vi "ReadIVBuffers.vi"(7 "GetCapacitors":bool, 8 "error in (no error)":errorcluster, 9 "Status":refnum<vi>, 10 "XYGraph Refnum":refnum<vi>, 11 "VISA Refnum in":refnum<visa-resource-name>) -> (0 "error out":errorcluster, 2 "CapacitanceInfos":T1[](array[typedef]), 3 "Array":dbl[][](array[numeric]))   [LabVIEW 2020]
uses:
  CapacitanceRecord.ctl
  Keithley 2600 Series/Keithley 2600 Series.lvlib
panel:
  out "Array 2":string[](array[string])
  out "error out 2":errorcluster
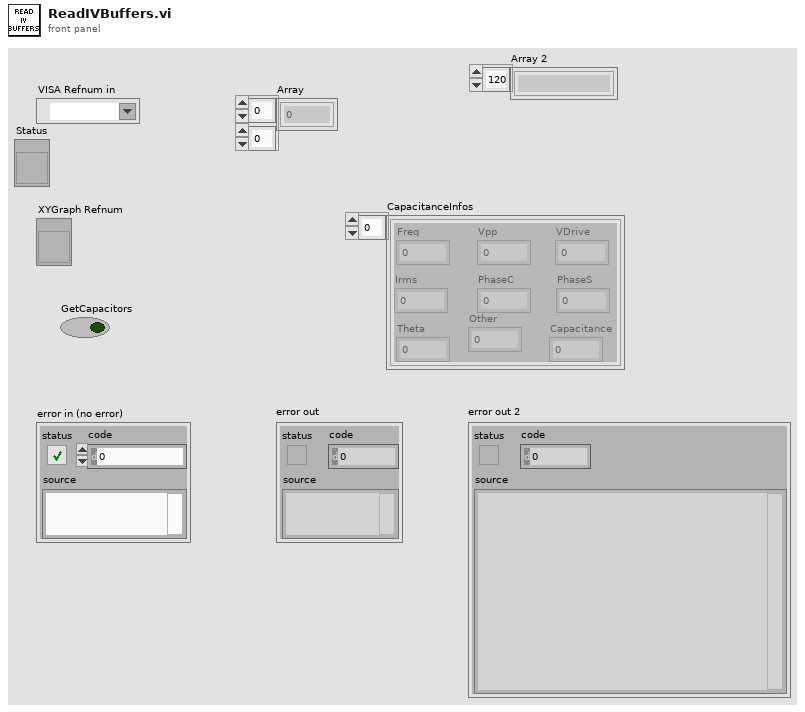
[diagram p1: front panel]
types:
  T1 = typedef "CapacitanceRecord.ctl" = cluster{"Freq":dbl, "Vpp":dbl, "PhaseS":dbl, "Irms":dbl, "PhaseC":dbl, "Theta":dbl, "VDrive":dbl, "Capacitance":dbl, "Other":dbl}
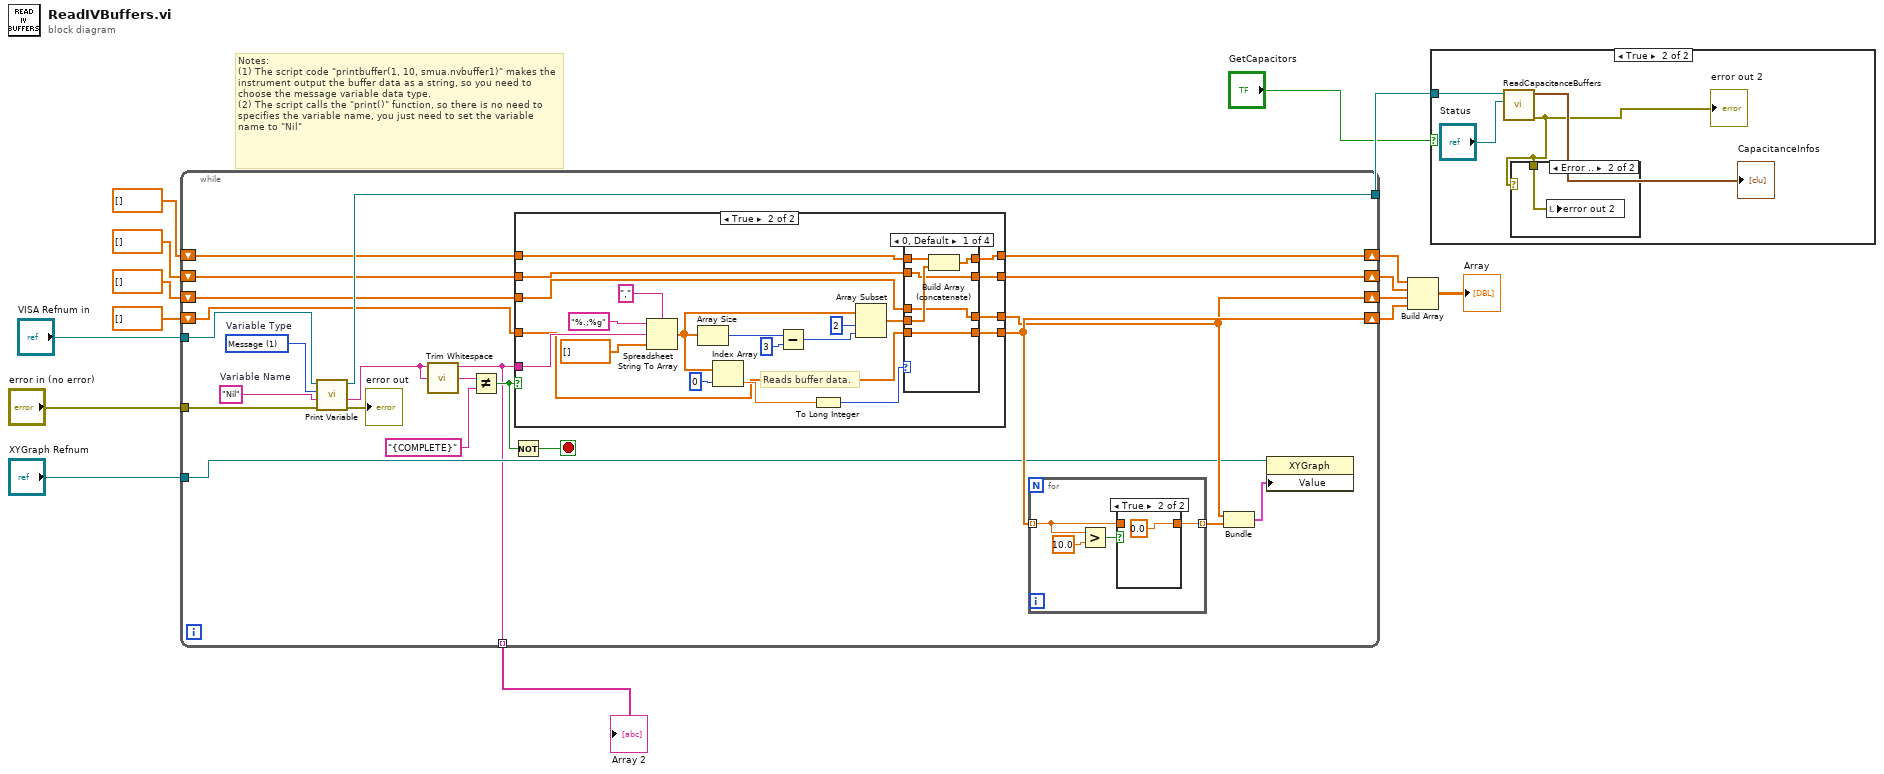
[diagram p0: block diagram]
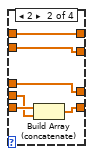
[diagram p6: hidden frame]
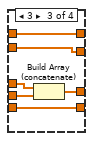
[diagram p7: hidden frame]
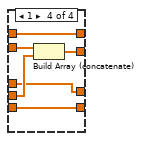
[diagram p8: hidden frame]
diagram:
  # "Notes: \n(1) The script code \"printbuffer(1, 10, smua.nvbuffer1)\" makes the instrument output the buffer data as a string, so you need to choose the message variable data type.\n(2) The script calls the \"print()\" function, so there is no need to specifies the variable name, you just need to set the variable name to \"Nil\""
  n1 = while {
    tunnel: "VISA Refnum in" -> [w35]
    tunnel: [w33] -> w3
    shift-right: [w28] -> w10
    shift-left: dbl[] [] ("array type (2D Dbl)") -> [w29]
    shift-right: [w18] -> w12
    shift-left: dbl[] [] ("array type (2D Dbl)") -> [w27]
    shift-right: [w32] -> w9
    shift-left: dbl[] [] ("array type (2D Dbl)") -> [w31]
    shift-right: [w19] -> w13
    shift-left: dbl[] [] ("array type (2D Dbl)") -> [w30]
    tunnel: "error in (no error)" -> [w22]
    tunnel: "XYGraph Refnum" -> [w17]
    tunnel: [w16] -> w1 mode=indexing
    stop <- w23 stop-if-true
    w37 = 1 items=["Number", "Message"]  # Variable Type
    w36 = "Nil"  # Variable Name
    n2 = call "Print Variable.vi"("error in (no error)"=w22, "Variable Name"=w36, "Variable Type (0: Number)"=w37, "VISA resource name"=w35) -> ("error out"=→"error out":errorcluster, "Message"=w16:string, "VISA resource name out"=w33:refnum<visa-resource-name>)  [unwired: 4 in, 1 out]
    n3 = call <vilib>:"Trim Whitespace.vi"("string"=w16) -> ("trimmed string"=w26:string)  [unwired: 1 in]
    n4 = Not Equal?(x=w26, y="{COMPLETE}") -> (x != y?=w24:bool)
    n5 = Not(x=w24) -> (.not. x?=w23:bool)
    n6 = case shown="True" w24 {
      tunnel: w16 -> [_ w65]
      tunnel: [w47 w63] -> w32
      tunnel: w31 -> [w47 w62]
      tunnel: [w45 w60] -> w19
      tunnel: w30 -> [w45 w58]
      tunnel: w29 -> [w46 w57]
      tunnel: [w46 w56] -> w28
      tunnel: w27 -> [w44 w55]
      tunnel: [w44 w54] -> w18
      frame False {
      }
      frame True {
        # "Reads buffer data."
        n7 = Spreadsheet String To Array(delimiter (Tab)=",", format string="%.;%g", spreadsheet string=w65, array type (2D Dbl)=dbl[] []) -> (array=w51:dbl[])
        n8 = Array Size(array=w51) -> (size(s)=w50:i32)
        n9 = Index Array(array=w51, index=0) -> (element=w61:dbl)
        n10 = Subtract(x=w50, y=3) -> (x-y=w48:i32)
        n11 = To Long Integer(number=w61) -> (32bit integer=w59:i32)
        n12 = Array Subset(array=w51, index=2, length=w48) -> (w53:dbl[])
        n13 = case shown="0, Default" w59 {
          tunnel: [w72 w80 w86 w92] -> w63
          tunnel: w62 -> [w74 w80 w86 w92]
          tunnel: [w71 w75 w85 w88] -> w60
          tunnel: w53 -> [w73 w78 w82 w90]
          tunnel: w58 -> [w71 w79 w85 w88]
          tunnel: w57 -> [w70 w77 w84 w91]
          tunnel: [w70 w77 w84 w89] -> w56
          tunnel: w55 -> [w69 w76 w83 w87]
          tunnel: [w69 w76 w81 w87] -> w54
          frame 0, Default {
            n14 = Build Array (concatenate)(w74, w73) -> (w72:dbl[])
          }
          frame 2 {
            n15 = Build Array (concatenate)(w79, w78) -> (w75:dbl[])
          }
          frame 3 {
            n16 = Build Array (concatenate)(w83, w82) -> (w81:dbl[])
          }
          frame 1 {
            n17 = Build Array (concatenate)(w91, w90) -> (w89:dbl[])
          }
        }
      }
    }
    n18 = for {
      tunnel: w19 -> [w39] mode=indexing
      tunnel: [w40] -> w20 mode=indexing
      n19 = Greater?(x=w39, y=10.0) -> (0:w41:bool)
      n20 = case shown="True" w41 {
        tunnel: [w42 0.0] -> w40
        tunnel: w39 -> [w42 _]
        frame False {
        }
        frame True {
        }
      }
    }
    n21 = Bundle("array type (2D Dbl)"=w18, w20) -> (w21:cluster{"array type (2D Dbl)":dbl[], dbl[]})  [unwired: 1 in]
    n22 = property class="XYGraph"(reference=w17, "Value"=w21) -> ()  [unwired: 1 in, 2 out]
  }
  "Array 2" <- w1
  n23 = Build Array(w9, w10, w12, w13) -> (→"Array":dbl[][])
  n24 = case shown="True" "GetCapacitors" {
    tunnel: w3 -> [_ w96]
    frame False {
    }
    frame True {
      n25 = call "ReadCapacitanceBuffers.vi"("Status"="Status", "VISA Refnum in"=w96) -> ("error out"=w93:errorcluster, "CapacitanceInfos"=→"CapacitanceInfos":T1[])  [unwired: 8 in]
      "error out 2" <- w93
      n26 = case shown="Error .." w93 {
        tunnel: w93 -> [_ w97]
        frame No Error {
        }
        frame Error {
          n27 = local write "error out 2"(w97) -> ()
        }
      }
    }
  }
